vi "AlmostEqual.vi"() -> ()   [LabVIEW 2016, in "DronaTest.lvlib" / "test_AssertControlValue.lvlib"]
uses:
  test_AssertControlValue.lvlib
  main/apis/Setup/GetVI/GetVIByPath.vi
  main/apis/Stimulus/ValueSignal/ValueSignalByPathString.vi
  main/Drona.lvlib
  main/apis/Stimulus/ValueSignal/ValueSignal.lvlib
  main/apis/Setup/GetVI/GetVI.lvlib
  <vilib>/addons/_JKI Toolkits/Caraya/classes/Test/Test.lvclass
  main/apis/Assert/AssertControlValue/AssertControlValue.lvlib
panel:
  out "error out":errorcluster
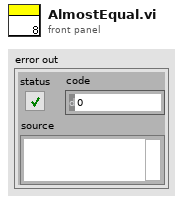
[diagram p1: front panel]
types:
  T1 = enum32{"Invalid", "Standard", "Closed", "Hidden", "Minimized", "Maximized"}
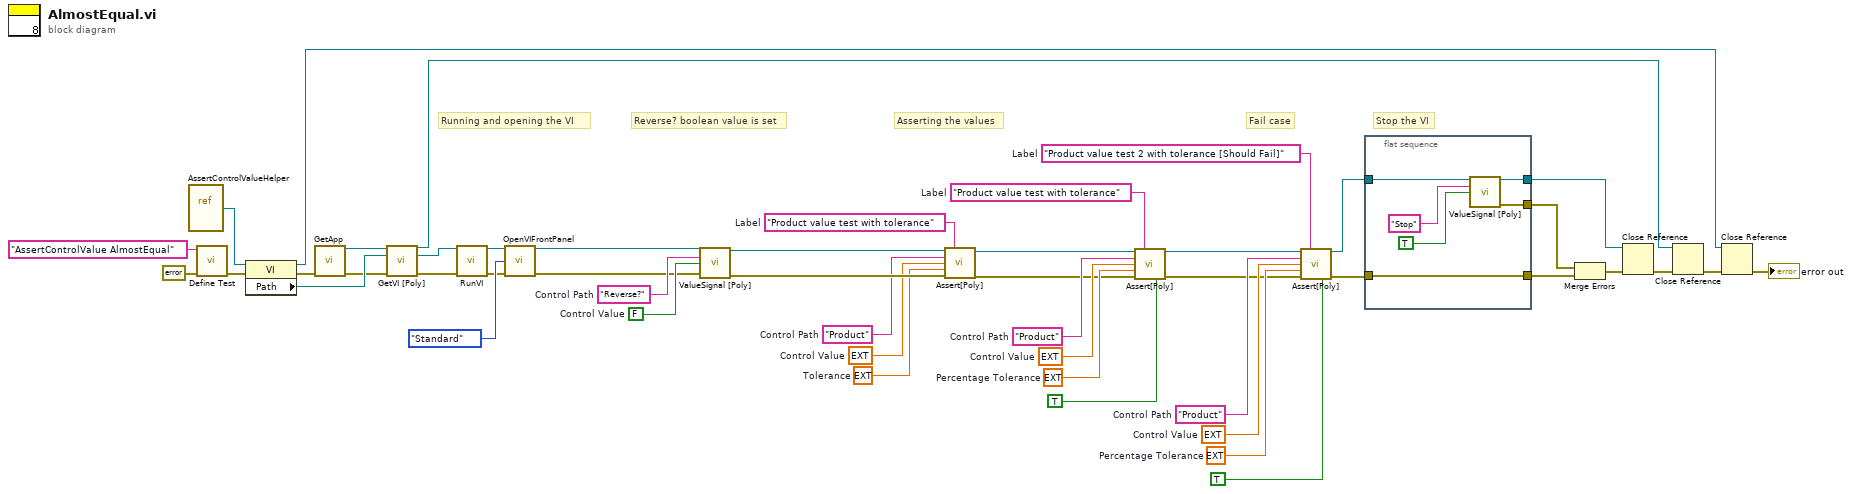
[diagram p0: block diagram]
diagram:
  w5 = "Product value test 2 with tolerance [Should Fail]"  # Label
  w10 = ext 10.0  # Percentage Tolerance
  w11 = ext 120.0  # Control Value
  w12 = "Product"  # Control Path
  w17 = "Product value test with tolerance"  # Label
  w20 = ext 50.0  # Percentage Tolerance
  w19 = ext 120.0  # Control Value
  w18 = "Product"  # Control Path
  w21 = "Product value test with tolerance"  # Label
  w22 = ext 10.0  # Tolerance
  w23 = ext 105.0  # Control Value
  w34 = "Product"  # Control Path
  w43 = FALSE  # Control Value
  w44 = "Reverse?"  # Control Path
  # "Stop the VI"
  # "Asserting the values"
  # "Reverse? boolean value is set"
  # "Running and opening the VI"
  # "Fail case"
  n1 = vi-ref "AssertControlValueHelper.vi"() -> (w38:refnum<vi>)
  n2 = call <vilib>:"Define Test.vi"("error in (no error)"=errorcluster {"status"=FALSE, "code"=0, "source"=""}, "Label (VI Title)"="AssertControlValue AlmostEqual") -> ("error out"=w39:errorcluster)  [unwired: 9 in]
  n3 = property on="Property Node" class="VI"(reference=w38, error in=w39) -> (reference out=w1:refnum<vi>, error out=w47:errorcluster, "Path"=w46:path)
  n4 = call "GetApp.vi"("error in (no error)"=w47) -> ("Application Ref"=w48:refnum<vi>, "error out"=w45:errorcluster)  [unwired: 13 in]
  n5 = call-poly "GetVI [Poly].vi"("Application Ref in"=w48, "VI Path"=w46, "error in (no error)"=w45) -> ("Application Ref out"=w2:refnum<vi>, "VI Reference"=w42:refnum<vi>, "error out"=w41:errorcluster)  [unwired: 10 in]
  n6 = call "RunVI.vi"("VI Reference In"=w42, "error in"=w41) -> ("VI Reference Out"=w24:refnum<vi>, "error out"=w25:errorcluster)  [unwired: 12 in]
  n7 = call "OpenVIFrontPanel.vi"("VI Reference In"=w24, "State(Standard)"=T1."Standard", "error in"=w25) -> ("VI Reference Out"=w28:refnum<vi>, "error out"=w27:errorcluster)  [unwired: 11 in]
  n8 = call-poly "ValueSignal [Poly].vi"("VI Reference In"=w28, "Control Path"=w44, "Value (Signaling)"=w43, "error in"=w27) -> ("VI Reference Out"=w35:refnum<vi>, "error out"=w36:errorcluster)  [unwired: 10 in]
  n9 = call-poly "Assert[Poly].vi"("VI Reference In"=w35, "Label"=w21, "Control Path"=w34, "Control Value"=w23, "Tolerance"=w22, "Error In"=w36) -> ("VI Reference Out"=w15:refnum<vi>, "Error Out"=w16:errorcluster)  [unwired: 8 in]
  n10 = call-poly "Assert[Poly].vi"("VI Reference In"=w15, "Label"=w17, "Control Path"=w18, "Control Value"=w19, "Tolerance"=w20, "Error In"=w16, "Use Percentage of X (F)"=TRUE) -> ("VI Reference Out"=w9:refnum<vi>, "Error Out"=w8:errorcluster)  [unwired: 7 in]
  n11 = call-poly "Assert[Poly].vi"("VI Reference In"=w9, "Label"=w5, "Control Path"=w12, "Control Value"=w11, "Tolerance"=w10, "Error In"=w8, "Use Percentage of X (F)"=TRUE) -> ("VI Reference Out"=w6:refnum<vi>, "Error Out"=w7:errorcluster)  [unwired: 7 in]
  n12 = flat-sequence {
    tunnel: w6 -> [w52]
    tunnel: [w51] -> w33
    tunnel: w7 -> [w50]
    tunnel: [w50] -> w32
    tunnel: [w49] -> w29
    frame #0 {
      n13 = call-poly "ValueSignal [Poly].vi"("VI Reference In"=w52, "Control Path"="Stop" ("Class Name"), "Value (Signaling)"=TRUE) -> ("VI Reference Out"=w49:refnum<vi>, "error out"=w51:errorcluster)  [unwired: 11 in]
    }
  }
  n14 = Merge Errors(w33, w32) -> (w31:errorcluster)
  n15 = Close Reference(reference=w29, error in (no error)=w31) -> (error out=w30:errorcluster)
  n16 = Close Reference(reference=w2, error in (no error)=w30) -> (error out=w4:errorcluster)
  n17 = Close Reference(reference=w1, error in (no error)=w4) -> (error out=→"error out":errorcluster)
